vi "Stop Core.vi"(10 "final error code":i32, 11 "KIT-QVA in":refnum<class "KIT-QVA.lvclass">) -> (3 "KIT-QVA out":refnum<class "KIT-QVA.lvclass">)   [LabVIEW 2014, in "KIT-QVA.lvlib" / "KIT-QVA.lvclass"]
doc: "(<B>Filename</B>: Actor Framework.lvlib:Actor.lvclass:Stop Core.vi)\n\nDefines what the actor does before it stops. Use the <B>final error code</B> input to determine whether the actor shut down in response to an error.\n\nBy default, this method does nothing. A descendant class may override it to define behavior, such as shutting down any processes the actor initiated in its override of the Actor Core method."
uses:
  KIT-QVA.lvclass
  KIT-QVA.lvclass/KIT-QVA.ctl
  CSPP_Core/Actors/CS++DeviceActor/CS++DeviceActor.lvclass
  CSPP_Core/Classes/CS++ProcessVariables/PVConnection/PVConnection.lvclass
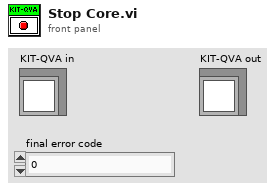
[diagram p1: front panel]
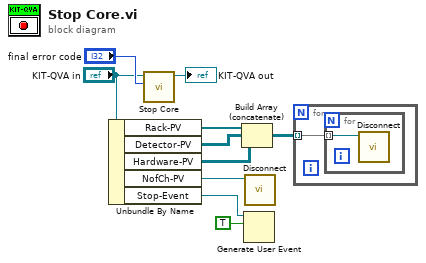
[diagram p0: block diagram]
diagram:
  n1 = Unbundle By Name("KIT-QVA in") -> ("Rack-PV"=w7:refnum<class "PVConnection.lvclass">[], "Detector-PV"=w6:refnum<class "PVConnection.lvclass">[][], "Hardware-PV"=w5:refnum<class "PVConnection.lvclass">[][], "NofCh-PV"=w3:refnum<class "PVConnection.lvclass">, "Stop-Event"=w2:refnum<user-event>)
  n2 = call-parent "Stop Core.vi"("final error code"="final error code", "CS++DeviceActor in"="KIT-QVA in") -> ("CS++DeviceActor out"=→"KIT-QVA out":refnum<class "KIT-QVA.lvclass">)  [unwired: 9 in]
  n3 = Build Array (concatenate)(w7, w6, w5) -> (w4:refnum<class "PVConnection.lvclass">[][])
  n4 = Generate User Event(user event=w2, event data cluster=TRUE ("event data")) -> ()  [unwired: 2 in, 2 out]
  n5 = call "Disconnect.vi"("PVConnection in"=w3) -> ()  [unwired: 9 in, 2 out]
  n6 = for {
    tunnel: w4 -> [w11] mode=indexing
    n7 = for {
      tunnel: w11 -> [w12] mode=indexing
      n8 = call "Disconnect.vi"("PVConnection in"=w12) -> ()  [unwired: 9 in, 2 out]
    }
  }
